vi "Generate Arc Maps.vi"(4 "Auto Release Stop Angle (Enabled)":bool=TRUE, 6 "Auto Release Start Angle (Enabled)":bool=TRUE, 7 "Auto Release Amount of Lines (Enabled)":bool=TRUE, 8 "error in (no error)":errorcluster, 9 "Stop Angle":refnum<class "1D Array f32.lvclass">, 10 "Start Angle":refnum<class "1D Array f32.lvclass">, 11 "Amount of Lines":refnum<class "1D Array s32.lvclass">) -> (0 "error out":errorcluster, 1 "Keys":refnum<class "2D Array u32.lvclass">, 2 "Point mask within bounds":refnum<class "2D Array binary.lvclass">, 3 "Arc Scales":refnum<class "2D Array f32.lvclass">)   [LabVIEW 2024, in "G2CPU Line Profile.lvlib"]
uses:
  G2CPU Line Profile.lvlib
  <vilib>/Natan Biesmans/G2CPU GPU and CPU HPC Toolkit/G2CPU Libraries/Arrays/1DArray/s32/1D Array s32.lvclass
  C:/Program Files/National Instruments/LabVIEW 2025/vi.lib/Natan Biesmans/G2CPU GPU and CPU HPC Toolkit/G2CPU Libraries/Arrays/Array/Array Prototype.lvclass
  <vilib>/Natan Biesmans/G2CPU GPU and CPU HPC Toolkit/G2CPU Libraries/Arrays/2DArray/binary/2D Array binary.lvclass
  <vilib>/Natan Biesmans/G2CPU GPU and CPU HPC Toolkit/G2CPU Libraries/Arrays/2DArray/u32/2D Array u32.lvclass
  <vilib>/Natan Biesmans/G2CPU GPU and CPU HPC Toolkit/G2CPU Libraries/Arrays/2DArray/f32/2D Array f32.lvclass
  <vilib>/Natan Biesmans/G2CPU GPU and CPU HPC Toolkit/G2CPU Libraries/Arrays/1DArray/f32/1D Array f32.lvclass
  6f650a5c-450f-4904-9550-55e0b3a4a5ae.vi
  3d39dc0d-773d-4b19-860c-3892fd35749d.vi
  54eba49e-e781-4b30-9dcf-830e96b50e96.vi
  26e62e18-ab6e-4879-8b70-f0624f3bc321.vi
  82cde389-861a-4c14-be8e-3c415f34a831.vi
  0de50304-b68d-4c0e-9536-b99c105c8d9a.vi
  84c39095-5878-4695-8f16-ab590e48028f.vi
  d8e68034-97e9-4a2f-baf8-c4ee0ec62345.vi
  02fc8ad5-646d-41dc-a33e-dc349fff4475.vi
  63b5cda9-a671-437d-9bda-18fe4a5707c3.vi
  40383f75-a77b-4927-b7ad-bc044501c951.vi
  6f650a5c-450f-4904-9550-55e0b3a4a5ae.vi/1bf6e03b-eb75-45f6-9764-49dc38a3a024.vi
  6f650a5c-450f-4904-9550-55e0b3a4a5ae.vi/2da4419f-02df-47a7-be00-1b7e0871fa33.vi
  3d39dc0d-773d-4b19-860c-3892fd35749d.vi/72eb0651-ae32-4ba2-a447-070823507cb2.vi
  54eba49e-e781-4b30-9dcf-830e96b50e96.vi/e7247370-a01f-465a-ac0e-4dfefcb1bb87.vi
  54eba49e-e781-4b30-9dcf-830e96b50e96.vi/345e91f0-9a5e-4de4-af9c-133346717e4a.vi
  26e62e18-ab6e-4879-8b70-f0624f3bc321.vi/ab6cfe59-c8ad-4da3-839b-8d02ec9e015f.vi
  82cde389-861a-4c14-be8e-3c415f34a831.vi/ab6cfe59-c8ad-4da3-839b-8d02ec9e015f.vi
  0de50304-b68d-4c0e-9536-b99c105c8d9a.vi/cfed8f62-9c64-4dab-912e-5e7c21cb720b.vi
  84c39095-5878-4695-8f16-ab590e48028f.vi/5793b77b-c002-4ebf-9075-685617c95341.vi
  84c39095-5878-4695-8f16-ab590e48028f.vi/2ed3ef86-c00d-4d71-b84c-20267a6dfcf9.vi
  d8e68034-97e9-4a2f-baf8-c4ee0ec62345.vi/2cbae9c5-d993-4013-91e6-67de96abb5a0.vi
  d8e68034-97e9-4a2f-baf8-c4ee0ec62345.vi/df7b902d-6356-419a-b5d5-2ac54df1e506.vi
  02fc8ad5-646d-41dc-a33e-dc349fff4475.vi/46771f49-eb1d-473b-8e81-f516cef50a4e.vi
  02fc8ad5-646d-41dc-a33e-dc349fff4475.vi/dc76f8e4-64fa-456a-8549-7a4b6936c4c9.vi
  02fc8ad5-646d-41dc-a33e-dc349fff4475.vi/7e60ddfb-e748-4c0c-85da-e395a1b7978d.vi
  02fc8ad5-646d-41dc-a33e-dc349fff4475.vi/d2eceff7-f641-4ce4-acfa-e9e293a3c877.vi
  02fc8ad5-646d-41dc-a33e-dc349fff4475.vi/b737122b-4036-448b-abd3-e2701355e828.vi
  63b5cda9-a671-437d-9bda-18fe4a5707c3.vi/6197f869-f6d4-49b3-9b2c-cc979b422c2e.vi
  63b5cda9-a671-437d-9bda-18fe4a5707c3.vi/a7e86dbb-b4c0-485c-89c5-522e60ee265c.vi
  40383f75-a77b-4927-b7ad-bc044501c951.vi/5793b77b-c002-4ebf-9075-685617c95341.vi
  40383f75-a77b-4927-b7ad-bc044501c951.vi/2ed3ef86-c00d-4d71-b84c-20267a6dfcf9.vi
  6f650a5c-450f-4904-9550-55e0b3a4a5ae.vi/1bf6e03b-eb75-45f6-9764-49dc38a3a024.vi/3e802c67-fb96-46a3-ae13-4994a8508b4f.vi
  6f650a5c-450f-4904-9550-55e0b3a4a5ae.vi/1bf6e03b-eb75-45f6-9764-49dc38a3a024.vi/5a50fc67-79e7-4972-80c2-92243cd53dd4.vi
  6f650a5c-450f-4904-9550-55e0b3a4a5ae.vi/2da4419f-02df-47a7-be00-1b7e0871fa33.vi/730f6c57-5c0b-4ee9-b61e-75067b25222b.vi
  6f650a5c-450f-4904-9550-55e0b3a4a5ae.vi/2da4419f-02df-47a7-be00-1b7e0871fa33.vi/096b8799-7810-404e-baca-ba9279cec4bd.vi
  6f650a5c-450f-4904-9550-55e0b3a4a5ae.vi/2da4419f-02df-47a7-be00-1b7e0871fa33.vi/0f1a5a47-bcc5-4796-ac31-8dfcfbc0d7d1.vi
  6f650a5c-450f-4904-9550-55e0b3a4a5ae.vi/2da4419f-02df-47a7-be00-1b7e0871fa33.vi/89f12e17-3330-4b72-ad8f-8dd636660732.vi
  26e62e18-ab6e-4879-8b70-f0624f3bc321.vi/ab6cfe59-c8ad-4da3-839b-8d02ec9e015f.vi/313ec8c5-c203-475c-9de0-0583f6fb8b4d.vi
  82cde389-861a-4c14-be8e-3c415f34a831.vi/ab6cfe59-c8ad-4da3-839b-8d02ec9e015f.vi/313ec8c5-c203-475c-9de0-0583f6fb8b4d.vi
  0de50304-b68d-4c0e-9536-b99c105c8d9a.vi/cfed8f62-9c64-4dab-912e-5e7c21cb720b.vi/77c7badc-ed81-4514-99c1-20d37f4e5ecc.vi
  0de50304-b68d-4c0e-9536-b99c105c8d9a.vi/cfed8f62-9c64-4dab-912e-5e7c21cb720b.vi/eb76fa01-6782-47b4-b34f-9eb474c9cc78.vi
  84c39095-5878-4695-8f16-ab590e48028f.vi/5793b77b-c002-4ebf-9075-685617c95341.vi/3e802c67-fb96-46a3-ae13-4994a8508b4f.vi
  84c39095-5878-4695-8f16-ab590e48028f.vi/5793b77b-c002-4ebf-9075-685617c95341.vi/5a50fc67-79e7-4972-80c2-92243cd53dd4.vi
  84c39095-5878-4695-8f16-ab590e48028f.vi/2ed3ef86-c00d-4d71-b84c-20267a6dfcf9.vi/730f6c57-5c0b-4ee9-b61e-75067b25222b.vi
  84c39095-5878-4695-8f16-ab590e48028f.vi/2ed3ef86-c00d-4d71-b84c-20267a6dfcf9.vi/096b8799-7810-404e-baca-ba9279cec4bd.vi
  84c39095-5878-4695-8f16-ab590e48028f.vi/2ed3ef86-c00d-4d71-b84c-20267a6dfcf9.vi/0f1a5a47-bcc5-4796-ac31-8dfcfbc0d7d1.vi
  84c39095-5878-4695-8f16-ab590e48028f.vi/2ed3ef86-c00d-4d71-b84c-20267a6dfcf9.vi/89f12e17-3330-4b72-ad8f-8dd636660732.vi
  d8e68034-97e9-4a2f-baf8-c4ee0ec62345.vi/df7b902d-6356-419a-b5d5-2ac54df1e506.vi/edd31282-7992-4bba-af75-482693dee5e1.vi
  02fc8ad5-646d-41dc-a33e-dc349fff4475.vi/dc76f8e4-64fa-456a-8549-7a4b6936c4c9.vi/3e802c67-fb96-46a3-ae13-4994a8508b4f.vi
  02fc8ad5-646d-41dc-a33e-dc349fff4475.vi/dc76f8e4-64fa-456a-8549-7a4b6936c4c9.vi/5a50fc67-79e7-4972-80c2-92243cd53dd4.vi
  63b5cda9-a671-437d-9bda-18fe4a5707c3.vi/6197f869-f6d4-49b3-9b2c-cc979b422c2e.vi/3e802c67-fb96-46a3-ae13-4994a8508b4f.vi
  63b5cda9-a671-437d-9bda-18fe4a5707c3.vi/6197f869-f6d4-49b3-9b2c-cc979b422c2e.vi/5a50fc67-79e7-4972-80c2-92243cd53dd4.vi
  63b5cda9-a671-437d-9bda-18fe4a5707c3.vi/a7e86dbb-b4c0-485c-89c5-522e60ee265c.vi/730f6c57-5c0b-4ee9-b61e-75067b25222b.vi
  63b5cda9-a671-437d-9bda-18fe4a5707c3.vi/a7e86dbb-b4c0-485c-89c5-522e60ee265c.vi/096b8799-7810-404e-baca-ba9279cec4bd.vi
  63b5cda9-a671-437d-9bda-18fe4a5707c3.vi/a7e86dbb-b4c0-485c-89c5-522e60ee265c.vi/0f1a5a47-bcc5-4796-ac31-8dfcfbc0d7d1.vi
  63b5cda9-a671-437d-9bda-18fe4a5707c3.vi/a7e86dbb-b4c0-485c-89c5-522e60ee265c.vi/89f12e17-3330-4b72-ad8f-8dd636660732.vi
  40383f75-a77b-4927-b7ad-bc044501c951.vi/5793b77b-c002-4ebf-9075-685617c95341.vi/3e802c67-fb96-46a3-ae13-4994a8508b4f.vi
  40383f75-a77b-4927-b7ad-bc044501c951.vi/5793b77b-c002-4ebf-9075-685617c95341.vi/5a50fc67-79e7-4972-80c2-92243cd53dd4.vi
  40383f75-a77b-4927-b7ad-bc044501c951.vi/2ed3ef86-c00d-4d71-b84c-20267a6dfcf9.vi/730f6c57-5c0b-4ee9-b61e-75067b25222b.vi
  40383f75-a77b-4927-b7ad-bc044501c951.vi/2ed3ef86-c00d-4d71-b84c-20267a6dfcf9.vi/096b8799-7810-404e-baca-ba9279cec4bd.vi
  40383f75-a77b-4927-b7ad-bc044501c951.vi/2ed3ef86-c00d-4d71-b84c-20267a6dfcf9.vi/0f1a5a47-bcc5-4796-ac31-8dfcfbc0d7d1.vi
  40383f75-a77b-4927-b7ad-bc044501c951.vi/2ed3ef86-c00d-4d71-b84c-20267a6dfcf9.vi/89f12e17-3330-4b72-ad8f-8dd636660732.vi
  63b5cda9-a671-437d-9bda-18fe4a5707c3.vi/a7e86dbb-b4c0-485c-89c5-522e60ee265c.vi/730f6c57-5c0b-4ee9-b61e-75067b25222b.vi/0070e0fe-4ad7-4a3e-8965-d64becb7e5f0.vi
  40383f75-a77b-4927-b7ad-bc044501c951.vi/2ed3ef86-c00d-4d71-b84c-20267a6dfcf9.vi/730f6c57-5c0b-4ee9-b61e-75067b25222b.vi/0070e0fe-4ad7-4a3e-8965-d64becb7e5f0.vi
  <vilib>/Natan Biesmans/G2CPU GPU and CPU HPC Toolkit/G2CPU Libraries/Arrays/SubVI/Lock Arrays.vi
  <vilib>/Natan Biesmans/G2CPU GPU and CPU HPC Toolkit/G2CPU Libraries/Arrays/Array/G2CPU Get Array Pointer.vi
  <vilib>/Natan Biesmans/G2CPU GPU and CPU HPC Toolkit/G2CPU Libraries/Arrays/SubVI/is 1D.vi
  <vilib>/Natan Biesmans/G2CPU GPU and CPU HPC Toolkit/ArrayFire Driver/VIs/sub.vi
  <vilib>/Natan Biesmans/G2CPU GPU and CPU HPC Toolkit/G2CPU Libraries/Arrays/Array/G2CPU Set Array Pointer.vi
  <vilib>/Natan Biesmans/G2CPU GPU and CPU HPC Toolkit/G2CPU Libraries/Arrays/Array/G2CPU Unlock Array.vi
  <vilib>/Natan Biesmans/G2CPU GPU and CPU HPC Toolkit/G2CPU Libraries/Arrays/Array/G2CPU Release Array.vi
  <vilib>/Natan Biesmans/G2CPU GPU and CPU HPC Toolkit/G2CPU Libraries/Arrays/Array/G2CPU Lock Array.vi
  <vilib>/Natan Biesmans/G2CPU GPU and CPU HPC Toolkit/ArrayFire Driver/VIs/max all.vi
  <vilib>/Natan Biesmans/G2CPU GPU and CPU HPC Toolkit/ArrayFire Driver/VIs/cast.vi
  <vilib>/Natan Biesmans/G2CPU GPU and CPU HPC Toolkit/ArrayFire Driver/VIs/range.vi
  <vilib>/Natan Biesmans/G2CPU GPU and CPU HPC Toolkit/ArrayFire Driver/VIs/Run as Multi Device.vi
  <vilib>/Natan Biesmans/G2CPU GPU and CPU HPC Toolkit/ArrayFire Driver/VIs/iszero.vi
  <vilib>/Natan Biesmans/G2CPU GPU and CPU HPC Toolkit/ArrayFire Driver/VIs/release array.vi
  <vilib>/Natan Biesmans/G2CPU GPU and CPU HPC Toolkit/G2CPU Libraries/Manage Environment/Find AF DLL.vi
  <vilib>/Natan Biesmans/G2CPU GPU and CPU HPC Toolkit/ArrayFire Driver/subvi/Error Converter (ErrCode or Status).vi
  <vilib>/Natan Biesmans/G2CPU GPU and CPU HPC Toolkit/ArrayFire Driver/VIs/add.vi
  <vilib>/Natan Biesmans/G2CPU GPU and CPU HPC Toolkit/G2CPU Libraries/Arrays/SubVI/is 2D.vi
  <vilib>/Natan Biesmans/G2CPU GPU and CPU HPC Toolkit/ArrayFire Driver/VIs/lt.vi
  <vilib>/Natan Biesmans/G2CPU GPU and CPU HPC Toolkit/ArrayFire Driver/VIs/div.vi
  <vilib>/Natan Biesmans/G2CPU GPU and CPU HPC Toolkit/ArrayFire Driver/VIs/mul.vi
  <vilib>/Natan Biesmans/G2CPU GPU and CPU HPC Toolkit/G2CPU Libraries/Arrays/Array/Array Prototype.lvclass
  <vilib>/Natan Biesmans/G2CPU GPU and CPU HPC Toolkit/G2CPU Libraries/Arrays/DataTypes/f32/f32.lvclass
  <vilib>/Natan Biesmans/G2CPU GPU and CPU HPC Toolkit/G2CPU Libraries/Arrays/1DArray/1D Array Prototype.lvclass
  <vilib>/Natan Biesmans/G2CPU GPU and CPU HPC Toolkit/G2CPU Libraries/Arrays/2DArray/2D Array Prototype.lvclass
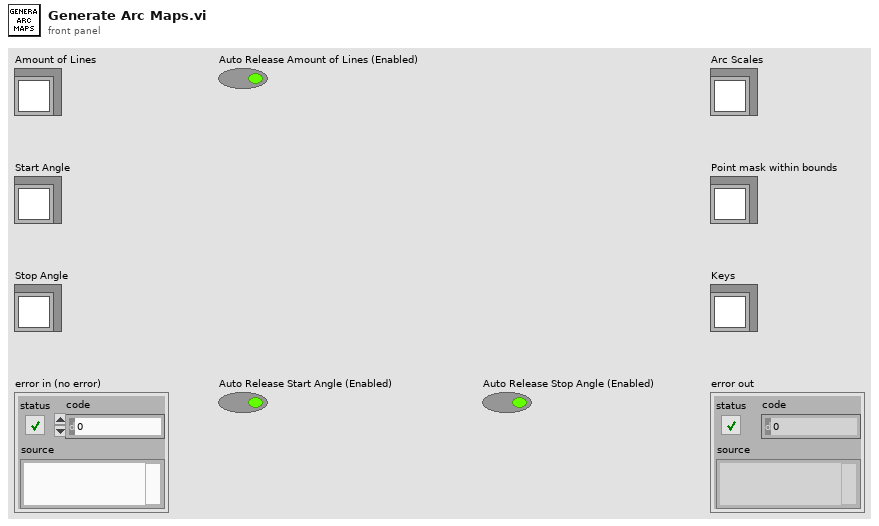
[diagram p1: front panel]
types:
  T1 = typedef "AF.lvlib/Dim4.ctl" = cluster{"Dim 0":u64, "Dim 1":u64, "Dim 2":u64, "Dim 3":u64}
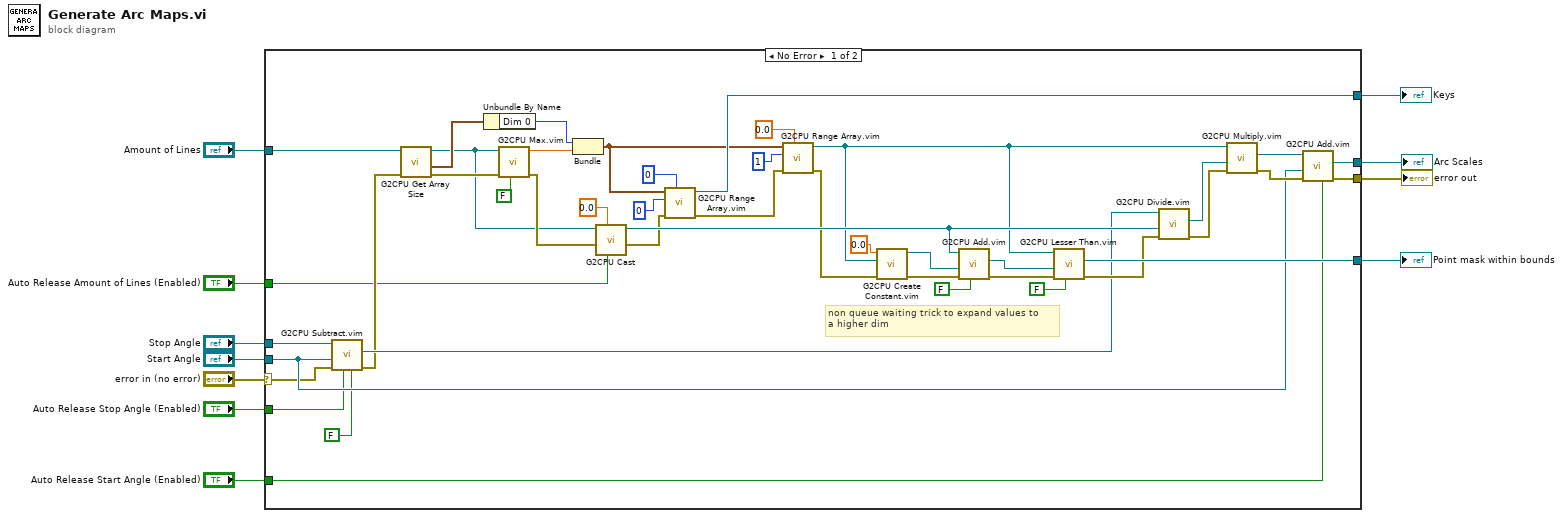
[diagram p0: block diagram]
diagram:
  n1 = case shown="No Error" "error in (no error)" {
    selector: "error in (no error)" -> [w18 w56]
    tunnel: "Amount of Lines" -> [w55 _]
    tunnel: [w54 _] -> w9
    tunnel: [w40 _] -> w8
    tunnel: [w22 _] -> w7
    tunnel: [w20 w56] -> w6
    tunnel: "Stop Angle" -> [w25 _]
    tunnel: "Start Angle" -> [w19 _]
    tunnel: "Auto Release Stop Angle (Enabled)" -> [w15 _]
    tunnel: "Auto Release Start Angle (Enabled)" -> [w13 _]
    tunnel: "Auto Release Amount of Lines (Enabled)" -> [w14 _]
    frame No Error {
      # "non queue waiting trick to expand values to\na higher dim"
      n2 = call "G2CPU Subtract.vim"("Auto Release rhs (Enabled)"=FALSE, "Auto Release lhs (Enabled)"=w15, "error in (no error)"=w18, "Array rhs"=w19, "Array lhs"=w25) -> ("error out"=w17:errorcluster, "Array Result"=w24:refnum<class "1D Array f32.lvclass">)  [unwired: 5 in]
      n3 = call <vilib>:"G2CPU Get Array Size.vi"("error in (no error)"=w17, "Array in"=w55) -> ("error out"=w42:errorcluster, "Array Size"=w43:T1, "Array out"=w16:refnum<class "1D Array s32.lvclass">)  [unwired: 6 in, 1 out]
      n4 = Unbundle By Name(w43) -> ("Dim 0"=w28:u64)
      n5 = call "G2CPU Max.vim"("Auto Release (Enabled)"=FALSE, "error in (no error)"=w42, "Array First"=w16) -> ("error out"=w33:errorcluster, "real out"=w29:dbl)  [unwired: 6 in, 1 out]
      n6 = Bundle("Dim 0"=w28, "real out"=w29) -> (w37:cluster{"Dim 0":u64, "real out":dbl})  [unwired: 1 in]
      n7 = call "G2CPU Cast"("Auto Release Low (Enabled)"=w14, "Datatype Prototype"=sgl 0.0 ("single precision float"), "error in (no error)"=w33, "Array In"=w16) -> ("error out"=w38:errorcluster, "Array Out"=w50:refnum<class "1D Array f32.lvclass">)  [unwired: 6 in]
      n8 = call "G2CPU Range Array.vim"("Datatype"=u32 0, "Error in"=w38, "Sequential Dimension"=0, "Size"=w37) -> ("error out"=w39:errorcluster, "Array out"=w40:refnum<class "2D Array u32.lvclass">)  [unwired: 6 in]
      n9 = call "G2CPU Range Array.vim"("Datatype"=sgl 0.0, "Error in"=w39, "Sequential Dimension"=1, "Size"=w37) -> ("error out"=w45:errorcluster, "Array out"=w46:refnum<class "2D Array f32.lvclass">)  [unwired: 6 in]
      n10 = call "G2CPU Create Constant.vim"("error in (no error)"=w45, "Size"=w46, "val"=sgl 0.0) -> ("error out"=w47:errorcluster, "object out"=w49:refnum<class "2D Array f32.lvclass">)  [unwired: 7 in]
      n11 = call "G2CPU Add.vim"("Auto Release lhs (Enabled)"=FALSE, "error in (no error)"=w47, "Array rhs"=w49, "Array lhs"=w50) -> ("error out"=w48:errorcluster, "Array Result"=w51:refnum<class "2D Array f32.lvclass">)  [unwired: 6 in]
      n12 = call "G2CPU Lesser Than.vim"("Auto Release lhs (Enabled)"=FALSE, "error in (no error)"=w48, "Array rhs"=w51, "Array lhs"=w46) -> ("error out"=w41:errorcluster, "Array Result"=w54:refnum<class "2D Array binary.lvclass">)  [unwired: 6 in]
      n13 = call "G2CPU Divide.vim"("error in (no error)"=w41, "Array rhs"=w50, "Array lhs"=w24) -> ("error out"=w31:errorcluster, "Array Result"=w34:refnum<class "1D Array f32.lvclass">)  [unwired: 7 in]
      n14 = call "G2CPU Multiply.vim"("error in (no error)"=w31, "Array rhs"=w34, "Array lhs"=w46) -> ("error out"=w21:errorcluster, "Array Result"=w23:refnum<class "2D Array f32.lvclass">)  [unwired: 7 in]
      n15 = call "G2CPU Add.vim"("Auto Release rhs (Enabled)"=w13, "error in (no error)"=w21, "Array rhs"=w19, "Array lhs"=w23) -> ("error out"=w20:errorcluster, "Array Result"=w22:refnum<class "2D Array f32.lvclass">)  [unwired: 6 in]
    }
    frame Error {
    }
  }
  "Point mask within bounds" <- w9
  "Keys" <- w8
  "Arc Scales" <- w7
  "error out" <- w6
